vi "_PC_Pub_ExpCondiValue_Script.vi"(2 "error in (no error)":errorcluster, 3 "expCondiVariant":variant) -> (0 "error out":errorcluster, 1 "scriptCode":string)   [LabVIEW 2018]
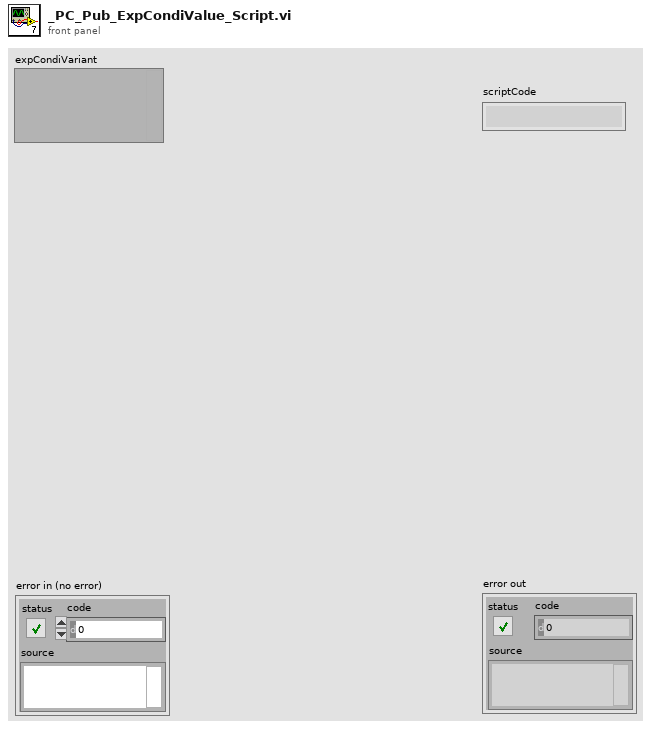
[diagram p1: front panel]
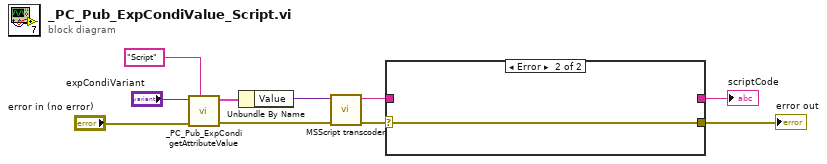
[diagram p0: block diagram]
diagram:
  n1 = call "_PC_Pub_ExpCondi getAttributeValue.vi"("attrName"="Script", "error in (no error)"="error in (no error)", "expCondiVariant"="expCondiVariant") -> ("error out"=w3:errorcluster, "attrValue"=w10:cluster{"Label":string, "Value":variant})  [unwired: 7 in]
  n2 = Unbundle By Name(w10) -> ("Value"=w5:variant)
  n3 = call "MSScript transcoder.vi"("error in (no error)"=w3, "new value"=w5) -> ("error out"=w2:errorcluster, "script code"=w4:string)  [unwired: 8 in]
  n4 = case shown="Error" w2 {
    selector: w2 -> [w11 w13]
    tunnel: w4 -> [w12 _]
    tunnel: [w12 _] -> w1
    tunnel: [w11 w13] -> w8
    frame No Error {
    }
    frame Error {
    }
  }
  "scriptCode" <- w1
  "error out" <- w8
